vi "Start TIRF Locked.vi"(8 "error in (no error)":errorcluster, 10 "TIRF Locked?":bool, 11 "DAQ_QPT_Throlab in":refnum<class "DAQ_QPT_Throlab.lvclass">) -> (0 "error out":errorcluster, 3 "DAQ_QPT_Throlab out":refnum<class "DAQ_QPT_Throlab.lvclass">)   [LabVIEW 2020, in "DAQ_QPT_Throlab.lvlib" / "DAQ_QPT_Throlab.lvclass"]
uses:
  DAQ_QPT_Throlab.lvclass
  DAQ_QPT_Throlab.lvclass/DAQ_QPT_Throlab.ctl
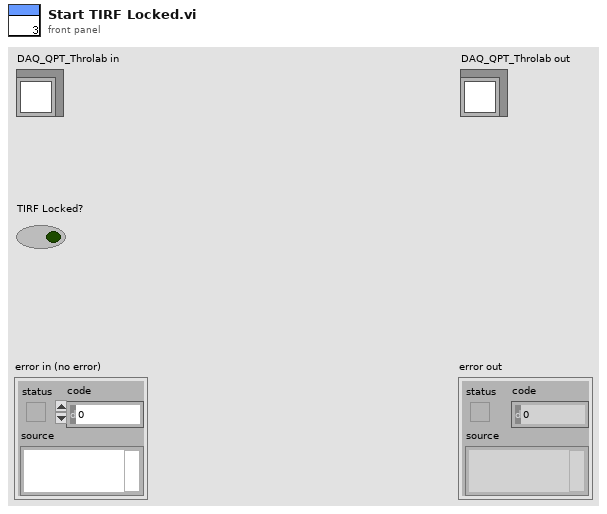
[diagram p1: front panel]
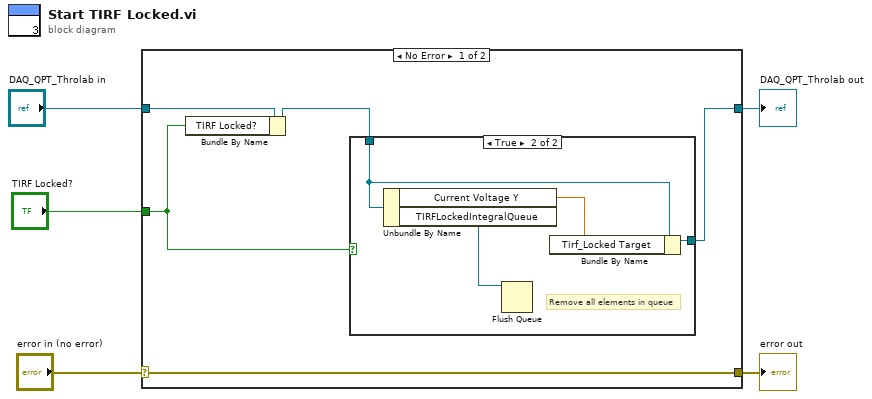
[diagram p0: block diagram]
diagram:
  n1 = case shown="No Error" "error in (no error)" {
    selector: "error in (no error)" -> [w10 w17]
    tunnel: [w10 w17] -> w4
    tunnel: [w6 w16] -> w2
    tunnel: "DAQ_QPT_Throlab in" -> [w9 w16]
    tunnel: "TIRF Locked?" -> [w8 _]
    frame No Error {
      n2 = Bundle By Name(cluster=w9, "TIRF Locked?"=w8) -> (w7:refnum<class "DAQ_QPT_Throlab.lvclass">)
      n3 = case shown="True" w8 {
        tunnel: w7 -> [w11 w14]
        tunnel: [w11 w15] -> w6
        frame False {
        }
        frame True {
          # "Remove all elements in queue"
          n4 = Unbundle By Name(w14) -> ("Current Voltage Y"=w13:dbl, "TIRFLockedIntegralQueue"=w12:refnum<queue>)
          n5 = Flush Queue(queue=w12) -> ()  [unwired: 1 in, 3 out]
          n6 = Bundle By Name(cluster=w14, "Tirf_Locked Target"=w13) -> (w15:refnum<class "DAQ_QPT_Throlab.lvclass">)
        }
      }
    }
    frame Error {
    }
  }
  "error out" <- w4
  "DAQ_QPT_Throlab out" <- w2
